vi "Write TMP PNG.vi"(8 "error in (no error)":errorcluster, 11 "img data":T1) -> (0 "error out":errorcluster, 3 "Base64 Encoded":string)   [LabVIEW 2024]
uses:
  <vilib>/picture/picture.llb/imagedata.ctl
  <vilib>/JDP Science/JDP Science Common Utilities/Base64/Base64 Support.lvlib
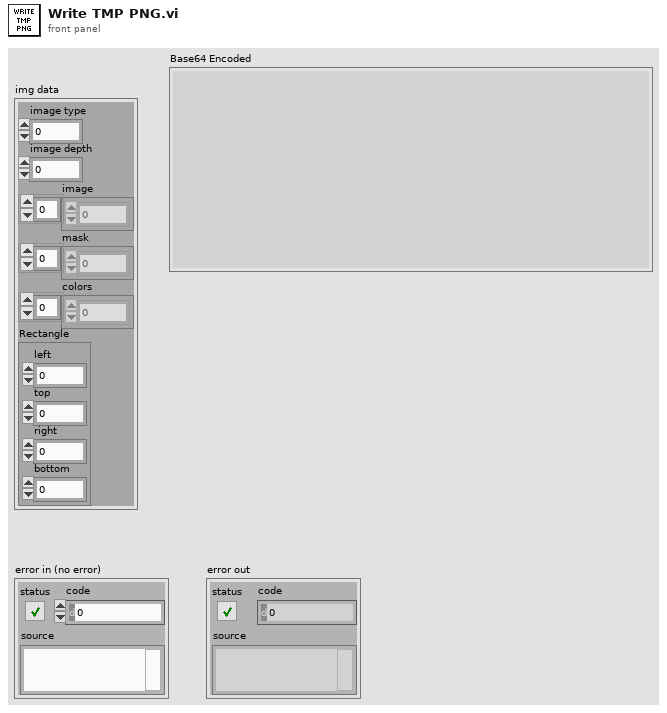
[diagram p1: front panel]
types:
  T1 = typedef "imagedata.ctl" = cluster{"image type":i32, "image depth":i32, "image":u8[], "mask":u8[], "colors":u32[], "Rectangle":cluster{"left":i16, "top":i16, "right":i16, "bottom":i16}}
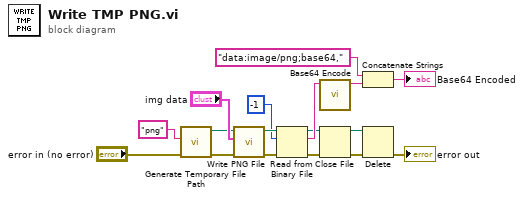
[diagram p0: block diagram]
diagram:
  n1 = call <vilib>:"Generate Temporary File Path.vi"("error in (no error)"="error in (no error)", "Temporary File Extension (tmp)"="png") -> ("error out"=w15:errorcluster, "Unique Temporary File Path"=w16:path)  [unwired: 8 in]
  n2 = call <vilib>:"Write PNG File.vi"("error in (no error)"=w15, "image data"="img data", "path to PNG file"=w16) -> ("error out"=w11:errorcluster, "path"=w10:path)  [unwired: 7 in]
  n3 = Read from Binary File(8:w11, 10:-1 ("count (1)"), 11:w10) -> (0:w8:errorcluster, 2:w12:string, 3:w6:refnum<file>)  [unwired: 3 in, 1 out]
  n4 = call <vilib>:"Base64 Encode.vi"("String to Encode"=w12) -> ("Base64 Encoded"=w2:string)  [unwired: 10 in]
  n5 = Close File(refnum=w6, error in=w8) -> (path=w5:path, error out=w7:errorcluster)
  n6 = Concatenate Strings("data:image/png;base64," ("string"), w2) -> (→"Base64 Encoded":string)
  n7 = Delete(path (use dialog)=w5, error in=w7) -> (error out=→"error out":errorcluster)  [unwired: 3 in, 2 out]
